vi "Nattify - Arrange FP Controls.vi"(0 "VI in":refnum<vi>, 1 "FP objects arrangement info":T1, 11 "error in":errorcluster) -> (4 "controls from conn pane":refnum<vi>[](array[refnum]), 6 "max bottom":i16, 15 "error out":errorcluster)   [LabVIEW 2020]
uses:
  Nattify - FP Objects Arrangement Info.ctl
  <vilib>/Utility/miscctls.llb/LVRectTypeDef.ctl
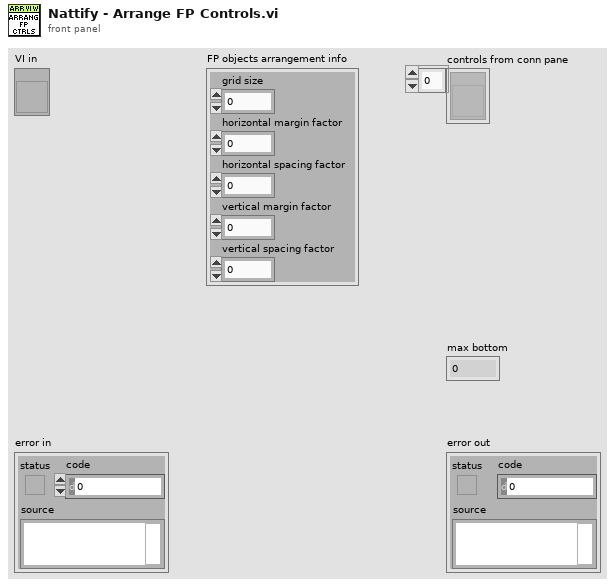
[diagram p1: front panel]
types:
  T1 = typedef "Nattify - FP Objects Arrangement Info.ctl" = cluster{"grid size":i32, "horizontal margin factor":i32, "horizontal spacing factor":i32, "vertical margin factor":i32, "vertical spacing factor":i32}
  T2 = enum32{"invalid VI type", "Standard VI", "Control VI", "Global VI", "Polymorphic VI", "Configuration VI", "SubSystem", "Facade VI", "Method VI", "Statechart Diagram VI"}
  T3 = typedef "LVRectTypeDef.ctl" = cluster{"Left":i16, "Top":i16, "Right":i16, "Bottom":i16}
  T4 = typedef "Nattify - FP Control Info.ctl" = cluster{"Terrminal Boundaries":T3, "Control Reference":refnum<vi>}
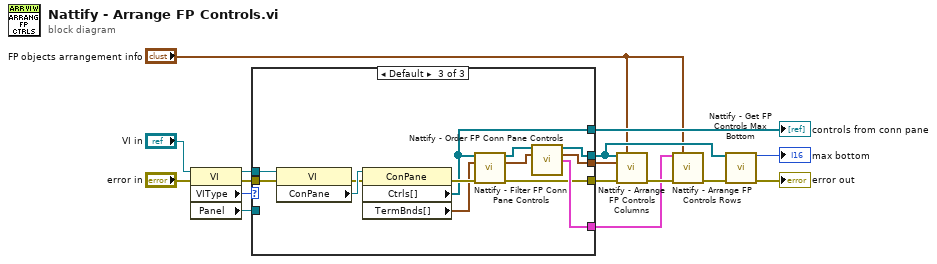
[diagram p0: block diagram]
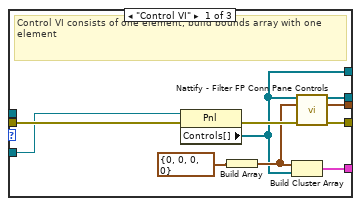
[diagram p2: hidden frame]
diagram:
  n1 = property class="VI"(reference="VI in", error in="error in") -> (reference out=w14:refnum<vi>, error out=w15:errorcluster, "VIType"=w16:T2, "Panel"=w11:refnum<vi>)
  n2 = case shown="Default" w16 {
    tunnel: [w20 _ w38] -> w7
    tunnel: [w21 _ w37] -> w6
    tunnel: [w22 w27 w32] -> w2
    tunnel: [w17 _ w34] -> w4
    tunnel: w14 -> [_ _ w36]
    tunnel: w15 -> [w24 w27 w35]
    tunnel: w11 -> [w23 _ _]
    tunnel: [w18 _ w28] -> w5
    frame "Control VI" {
      # "Control VI consists of one element; build bounds array with one element"
      n3 = property class="Pnl"(reference=w23, error in=w24) -> (error out=w25:errorcluster, "Controls[]"=w18:refnum<vi>[])  [unwired: 1 out]
      n4 = Build Array(T3 {"Left"=0, "Top"=0, "Right"=0, "Bottom"=0} ("Rectangle")) -> (w19:T3[])
      n5 = Build Cluster Array(w19, w18) -> (w17:cluster{"Rectangle":T3, refnum<vi>}[])
      n6 = call "Nattify - Filter FP Conn Pane Controls.vi"("controls in"=w18, "terminal boundaries"=w19, "error in"=w25) -> ("filtered controls"=w21:refnum<vi>[], "filtered terminal boundaries"=w20:T3[], "error out"=w22:errorcluster)  [unwired: 10 in]
    }
    frame "Global VI" {
      # "Don't arrange the controls of a global VI"
    }
    frame Default {
      n7 = property class="VI"(reference=w36, error in=w35) -> (error out=w39:errorcluster, "ConPane"=w40:refnum<vi>)  [unwired: 1 out]
      n8 = property class="ConPane"(reference=w40, error in=w39) -> (error out=w33:errorcluster, "Ctrls[]"=w28:refnum<vi>[], "TermBnds[]"=w31:T3[])  [unwired: 1 out]
      n9 = call "Nattify - Filter FP Conn Pane Controls.vi"("controls in"=w28, "terminal boundaries"=w31, "error in"=w33) -> ("filtered controls"=w30:refnum<vi>[], "filtered terminal boundaries"=w29:T3[], "error out"=w32:errorcluster)  [unwired: 10 in]
      n10 = call "Nattify - Order FP Conn Pane Controls.vi"("controls in"=w30, "terminal bounds"=w29) -> ("sorted controls"=w37:refnum<vi>[], "sorted terminal boundaries"=w38:T3[], "sorted array of control info"=w34:T4[])  [unwired: 11 in]
    }
  }
  "controls from conn pane" <- w5
  n11 = call "Nattify - Arrange FP Controls Columns.vi"("sorted controls"=w6, "FP objects arrangement info"="FP objects arrangement info", "sorted terminal boundaries"=w7, "error in"=w2) -> ("error out"=w12:errorcluster)  [unwired: 11 in]
  n12 = call "Nattify - Arrange FP Controls Rows.vi"("sorted array of control info"=w4, "FP objects arrangement info"="FP objects arrangement info", "error in"=w12) -> ("error out"=w10:errorcluster)  [unwired: 12 in]
  n13 = call "Nattify - Get FP Controls Max Bottom.vi"("controls"=w6, "error in"=w10) -> ("max bottom"=→"max bottom":i16, "error out"=→"error out":errorcluster)  [unwired: 12 in]
